vi "DAQmxSetupTiming.vi"(8 "error in (no error)":errorcluster, 10 "FsReq":dbl, 11 "TaskIn":refnum<k21>) -> (0 "error out":errorcluster, 2 "FsAchieved":dbl, 4 "bufferSizeAssigned":u32, 6 "totalPlannedSamples":i32)   [LabVIEW 2022 SP3]
uses:
  <vilib>/DAQmx/configure/timing.llb/DAQmx Timing (Sample Clock).vi
  Globals/Meas_global.vi
  <resource>/objmgr/daqmx.rc
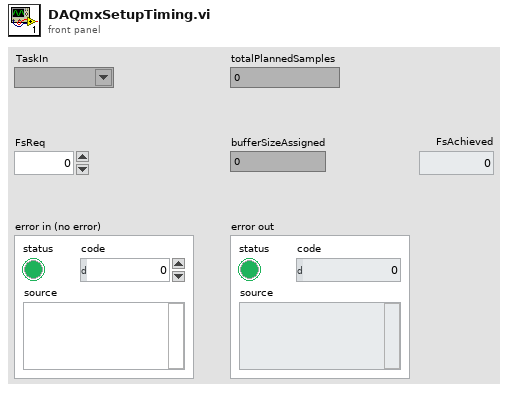
[diagram p1: front panel]
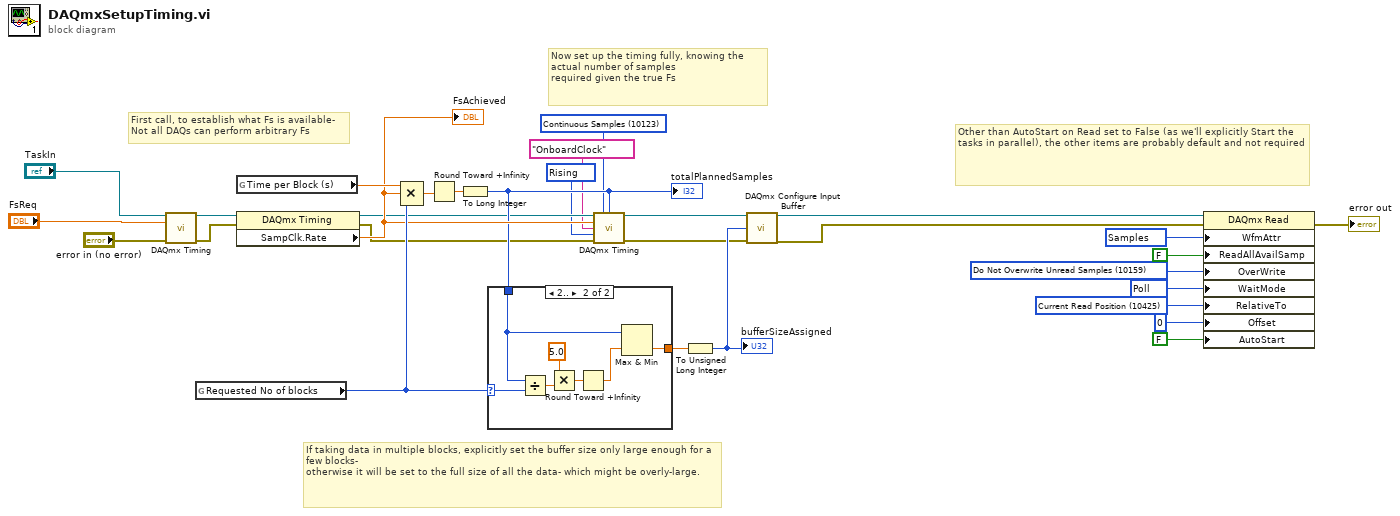
[diagram p0: block diagram]
diagram:
  w5 = 10425 items=["First Sample"=10424, "Current Read Position"=10425, "Reference Trigger"=10426, "First Pretrigger Sample"=10427, "Most Recent Sample"=10428] ("RelativeTo")
  w6 = 12524 items=["Wait For Interrupt"=12523, "Poll"=12524, "Yield"=12525, "Sleep"=12547] ("WaitMode")
  w7 = 10159 items=["Overwrite Unread Samples"=10252, "Do Not Overwrite Unread Samples"=10159] ("OverWrite")
  w9 = 10287 items=["Samples"=10287, "Samples and Timing"=10140, "Samples, Timing, and Attributes"=10141] ("WfmAttr")
  w17 = 10280 items=["Rising"=10280, "Falling"=10171] ("active edge")
  w15 = 10123 items=["Finite Samples"=10178, "Continuous Samples"=10123, "Hardware Timed Single Point"=12522] ("sample mode")
  # "Other than AutoStart on Read set to False (as we'll explicitly Start the tasks in parallel), the other items are probably default and not required"
  # "If taking data in multiple blocks, explicitly set the buffer size only large enough for a few blocks-\notherwise it will be set to the full size of all the data- which might be overly-large."
  # "Now set up the timing fully, knowing the actual number of samples\nrequired given the true Fs"
  # "First call, to establish what Fs is available-\nNot all DAQs can perform arbitrary Fs"
  n1 = call-poly <vilib>:"DAQmx Timing.vi"("task/channels in"="TaskIn", "rate"="FsReq", "error in"="error in (no error)") -> ("task out"=w14:refnum<k21>, "error out"=w19:errorcluster)  [unwired: 4 in, 7 out]
  n2 = global read "Meas_global.vi" "Requested No of blocks"() -> (w29:i32)
  n3 = global read "Meas_global.vi" "Time per Block (s)"() -> (w30:dbl)
  n4 = property class="DAQmx Timing"(reference=w14, error in=w19) -> (reference out=w18:refnum<k21>, error out=w20:errorcluster, "SampClk.Rate"=w27:dbl)
  "FsAchieved" <- w27
  n5 = Compound Arithmetic op=MULTIPLY(w30, w27, w29) -> (w28:dbl)
  n6 = Round Toward +Infinity(x=w28) -> (ceil(x): smallest int >= x=w21:dbl)
  n7 = To Long Integer(number=w21) -> (32bit integer=w22:i32)
  "totalPlannedSamples" <- w22
  n8 = case shown="2.." w29 {
    selector: w29 -> [_ w36]
    tunnel: w22 -> [w31 w34]
    tunnel: [w31 w32] -> w25
    frame 1, Default {
    }
    frame 2.. {
      n9 = Divide(x=w34, y=w36) -> (x/y=w38:dbl)
      n10 = Multiply(x=5.0, y=w38) -> (x*y=w35:dbl)
      n11 = Round Toward +Infinity(x=w35) -> (ceil(x): smallest int >= x=w33:dbl)
      n12 = Max & Min(x=w34, y=w33) -> (min(x,y)=w32:dbl)  [unwired: 1 out]
    }
  }
  n13 = call-poly <vilib>:"DAQmx Timing.vi"("task/channels in"=w18, "sample mode"=w15, "samples per channel"=w22, "rate"=w27, "source"=tag "OnboardClock", "active edge"=w17, "error in"=w20) -> ("task out"=w24:refnum<k21>, "error out"=w23:errorcluster)  [unwired: 7 out]
  n14 = To Unsigned Long Integer(number=w25) -> (unsigned 32bit integer=w26:u32)
  "bufferSizeAssigned" <- w26
  n15 = call <vilib>:"DAQmx Configure Input Buffer.vi"("task/channels in"=w24, "buffer size (in samples per channel)"=w26, "error in"=w23) -> ("task out"=w10:refnum<k21>, "error out"=w2:errorcluster)  [unwired: 11 in]
  n16 = property class="DAQmx Read"(reference=w10, error in=w2, "WfmAttr"=w9, "ReadAllAvailSamp"=FALSE, "OverWrite"=w7, "WaitMode"=w6, "RelativeTo"=w5, "Offset"=0, "AutoStart"=FALSE) -> (error out=→"error out":errorcluster)  [unwired: 1 out]
